vi "Destroy.vi"(8 "error in (no error)":errorcluster, 11 "reference in":refnum<class "A4.lvclass">) -> (0 "error out":errorcluster, 3 "reference out":refnum<class "A4.lvclass">)   [LabVIEW 2012, in "A4.lvclass"]
uses:
  A4.lvclass
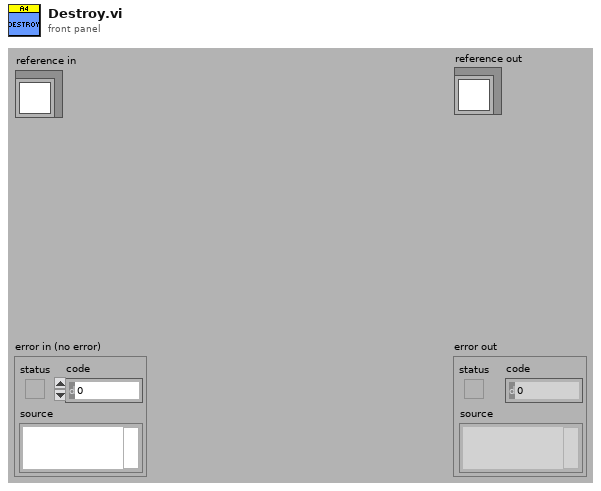
[diagram p1: front panel]
types:
  T1 = typedef "A4.lvclass/ObjectAttributes.ctl" = cluster{"Attribute1":dbl}
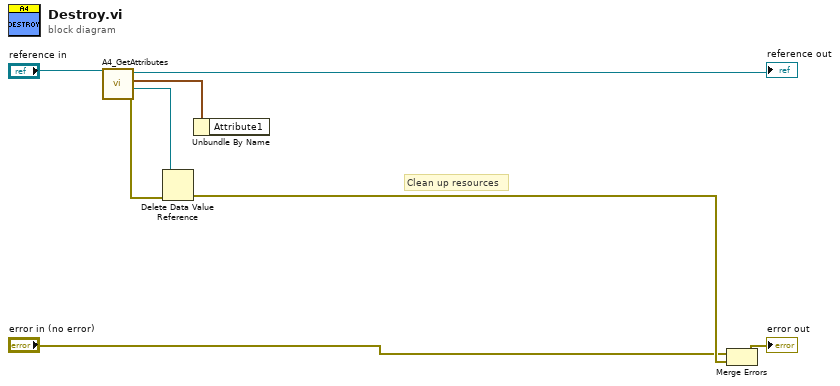
[diagram p0: block diagram]
diagram:
  # "Clean up resources"
  n1 = call "A4_GetAttributes.vi"("reference in"="reference in") -> ("error out"=w5:errorcluster, "DataRef"=w4:refnum<data-value>, "Data"=w3:T1, "reference out"=→"reference out":refnum<class "A4.lvclass">)  [unwired: 7 in]
  n2 = Delete Data Value Reference(data value reference=w4, error in=w5) -> (error out=w2:errorcluster)  [unwired: 1 out]
  n3 = Unbundle By Name(w3) -> ()  [unwired: 1 out]
  n4 = Merge Errors("error in (no error)", w2) -> (→"error out":errorcluster)
